vi "PopulatePads.vi"(0 "Set Pad?":bool, 1 "MeasureControl":refnum<vi>, 3 "Pad":string, 4 "PadArea":T1) -> ()   [LabVIEW 2012]
uses:
  Controls/PadArea.ctl
  Controls/MeasureControl.ctl
  Controls/TestData.ctl
  Controls/Measurement.ctl
  PadLookupVar.vi
panel:
  # "Measure Control"
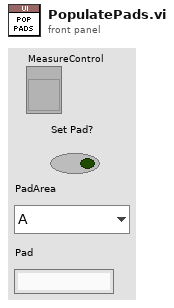
[diagram p1: front panel]
types:
  T1 = typedef "PadArea.ctl" = enum16{"A", "B", "C", "D", "L", "R", "T", "G"}
  T2 = typedef "PadLookup.ctl" = cluster{"A":T3, "B":T3, "C":T3, "D":T3, "L":T3, "R":T3, "T":T3, "G":T3}
  T3 = typedef "PadLookupItem.ctl" = cluster{"PadArea":T1, string[]}
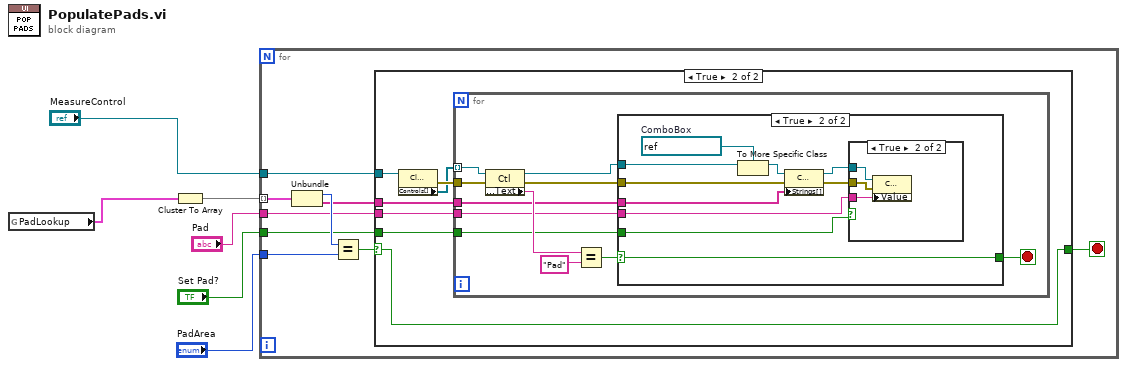
[diagram p0: block diagram]
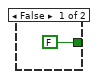
[diagram p3: hidden frame]
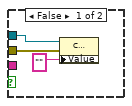
[diagram p4: hidden frame]
diagram:
  n1 = global read "PadLookupVar.vi" "PadLookup"() -> (w1:T2)
  n2 = Cluster To Array(cluster=w1) -> (array=w6:T3[])
  n3 = for {
    tunnel: w6 -> [w15] mode=indexing
    tunnel: "PadArea" -> [w10]
    tunnel: "MeasureControl" -> [w9]
    tunnel: "Set Pad?" -> [w8]
    tunnel: "Pad" -> [w7]
    stop <- w12 stop-if-true
    n4 = Unbundle(w15) -> ("PadArea"=w14:T1, w11:string[])
    n5 = Equal?(x=w14, y=w10) -> (x = y?=w13:bool)
    n6 = case shown="True" w13 {
      selector: w13 -> [w16 w23]
      tunnel: [w16 w23] -> w12
      tunnel: w11 -> [_ w19]
      tunnel: w9 -> [_ w20]
      tunnel: w8 -> [_ w18]
      tunnel: w7 -> [_ w17]
      frame False {
      }
      frame True {
        n7 = property class="Clust (strict)"(reference=w20) -> (error out=w22:errorcluster, "Controls[]"=w21:refnum<vi>[])  [unwired: 1 in, 1 out]
        n8 = for {
          tunnel: w21 -> [w34] mode=indexing
          tunnel: w19 -> [w29]
          tunnel: w22 -> [w27]
          tunnel: w18 -> [w25]
          tunnel: w17 -> [w24]
          stop <- w26 stop-if-true
          n9 = property class="Ctl"(reference=w34, error in=w27) -> (reference out=w30:refnum<vi>, error out=w28:errorcluster, "Label.Text"=w33:string)
          n10 = Equal?(x=w33, y="Pad") -> (x = y?=w31:bool)
          n11 = case shown="True" w31 {
            selector: w31 -> [_ w40]
            tunnel: w30 -> [_ w45]
            tunnel: w29 -> [_ w42]
            tunnel: w28 -> [_ w41]
            tunnel: [FALSE w40] -> w26
            tunnel: w25 -> [_ w39]
            tunnel: w24 -> [_ w36]
            frame False {
            }
            frame True {
              w44 = refnum<vi> refnum  # ComboBox
              n12 = To More Specific Class(target class=w44, reference=w45) -> (specific class reference=w43:refnum<vi>)  [unwired: 1 in, 1 out]
              n13 = property class="CmbBox"(reference=w43, error in=w41, "Strings[]"=w42) -> (reference out=w38:refnum<vi>, error out=w37:errorcluster)
              n14 = case shown="True" w39 {
                tunnel: w38 -> [w47 w51]
                tunnel: w37 -> [w46 w50]
                tunnel: w36 -> [_ w49]
                frame False {
                  n15 = property class="CmbBox"(reference=w47, error in=w46, "Value"="") -> ()  [unwired: 2 out]
                }
                frame True {
                  n16 = property class="CmbBox"(reference=w51, error in=w50, "Value"=w49) -> ()  [unwired: 2 out]
                }
              }
            }
          }
        }
      }
    }
  }
